vi "SNMP Encode SubID.vi"(8 "SubID String":u32) -> (1 "SubID Value":u32 format="%.0x", 2 "Encoded bits":bool[](array[boolean]), 3 "SubID byte array":u8[](array[numeric]) format="%.0x")   [LabVIEW 2017]
doc: "This VI is used to encode the value within the OID to the proper format as defined by the SNMP protocol. This is primarily used to decode OID values greater than 255."
panel:
  out "# of bytes in encoded ID":u8
  out "highest set bit":u8
  out "ID as Bit Array":bool[](array[boolean])
  # "*"
  # "*"
  # "*"
  # "*"
  # "*"
  # "*"
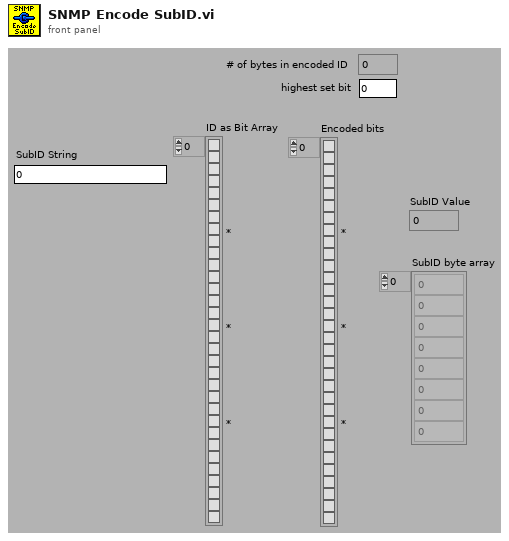
[diagram p1: front panel]
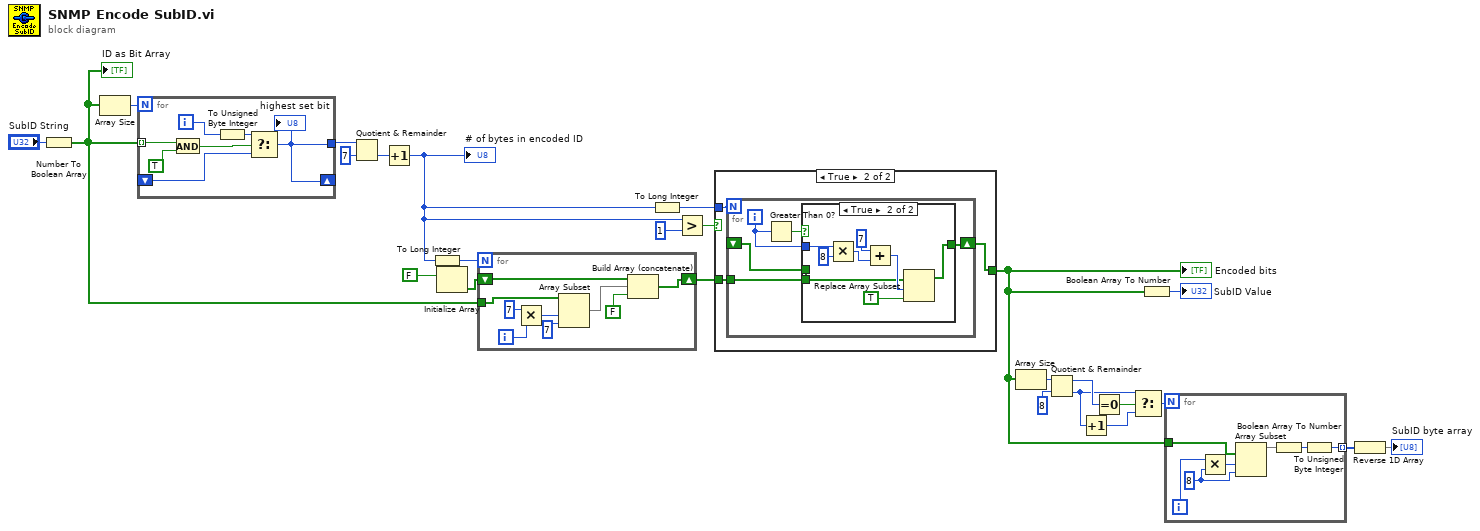
[diagram p0: block diagram]
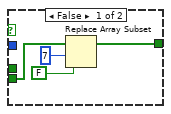
[diagram p3: hidden frame]
diagram:
  n1 = Number To Boolean Array(number="SubID String") -> (Boolean array=w21:bool[])
  "ID as Bit Array" <- w21
  n2 = Array Size(array=w21) -> (size(s)=w24:i32)
  n3 = for {
    N: w24 -> [_]
    tunnel: w21 -> [w32] mode=indexing
    tunnel: [w27] -> w23
    shift-right: [w27] -> _
    shift-left: _ -> [w28]
    i -> [w30]
    n4 = And(x=w32, y=TRUE) -> (x .and. y?=w29:bool)
    n5 = To Unsigned Byte Integer(number=w30) -> (unsigned 8bit integer=w26:u8)
    n6 = Select(t=w26, s=w29, f=w28) -> (s? t:f=w27:u8)
    "highest set bit" <- w27
  }
  n7 = Quotient & Remainder(x=w23, y=u8 7) -> (floor(x/y)=w16:u8)  [unwired: 1 out]
  n8 = Increment(x=w16) -> (x+1=w15:u8)
  "# of bytes in encoded ID" <- w15
  n9 = To Long Integer(number=w15) -> (32bit integer=w1:i32)
  n10 = Initialize Array(FALSE) -> (w20:bool[])  [unwired: 1 out]
  n11 = for {
    N: w1 -> [_]
    tunnel: w21 -> [w41]
    shift-right: [w33] -> w18
    shift-left: w20 -> [w36]
    i -> [w35]
    n12 = Multiply(x=7 ("y"), y=w35) -> (x*y=w39:i32)
    n13 = Array Subset(array=w41, index=w39, length=7) -> (w38:bool[])
    n14 = Build Array (concatenate)(w36, w38, FALSE) -> (w33:bool[])
  }
  n15 = To Long Integer(number=w15) -> (32bit integer=w2:i32)
  n16 = Greater?(x=w15, y=u8 1) -> (0:w13:bool)
  n17 = case shown="True" w13 {
    tunnel: w18 -> [w42 w45]
    tunnel: [w42 w43] -> w3
    tunnel: w2 -> [_ w44]
    frame False {
    }
    frame True {
      n18 = for {
        N: w44 -> [_]
        tunnel: w45 -> [w50]
        shift-right: [w46] -> w43
        shift-left: _ -> [w47]
        i -> [w48]
        n19 = Greater Than 0?(x=w48) -> (x > 0?=w49:bool)
        n20 = case shown="True" w49 {
          tunnel: w50 -> [w52 _]
          tunnel: [w51 w59] -> w46
          tunnel: w48 -> [_ w57]
          tunnel: w47 -> [_ w55]
          frame False {
            n21 = Replace Array Subset(array=w52, new element=FALSE, index=7 ("y")) -> (w51:bool[])
          }
          frame True {
            n22 = Multiply(x=w57, y=8) -> (x*y=w61:i32)
            n23 = Add(x=7, y=w61) -> (x+y=w58:i32)
            n24 = Replace Array Subset(array=w55, new element=TRUE, index=w58) -> (w59:bool[])
          }
        }
      }
    }
  }
  "Encoded bits" <- w3
  n25 = Array Size(array=w3) -> (size(s)=w12:i32)
  n26 = Quotient & Remainder(x=w12, y=8) -> (x-y*floor(x/y)=w10:i32, floor(x/y)=w8:i32)
  n27 = Increment(x=w8) -> (x+1=w7:i32)
  n28 = Equal To 0?(x=w10) -> (x = 0?=w9:bool)
  n29 = Select(t=w8, s=w9, f=w7) -> (s? t:f=w6:i32)
  n30 = Boolean Array To Number(Boolean array=w3) -> (number=→"SubID Value":u32)
  n31 = for {
    N: w6 -> [_]
    tunnel: w3 -> [w66]
    tunnel: [w63] -> w5 mode=indexing
    i -> [w69]
    w67 = 8
    n32 = Multiply(x=w69, y=w67) -> (x*y=w68:i32)
    n33 = Array Subset(array=w66, index=w68, length=w67) -> (w65:bool[])
    n34 = Boolean Array To Number(Boolean array=w65) -> (number=w64:u32)
    n35 = To Unsigned Byte Integer(number=w64) -> (unsigned 8bit integer=w63:u8)
  }
  n36 = Reverse 1D Array(array=w5) -> (reversed array=→"SubID byte array":u8[])
